vi "Keithley2400_TestReadout&Reset.vi"() -> ()   [LabVIEW 2018]
uses:
  <instrlib>/Keithley 24XX/Public/Data/Read (Single Point).vi
  <instrlib>/Keithley 24XX/Keithley 24XX.lvlib
panel:
  in  "Reset (Note, you  may need to set TRUE to get readout working! \nDon't use TRUE when measuring a device!). This program should loop\nthe voltage from the sourcemeter from 0V to 0.5V then jump to 0V and repeat.":bool
  in  "stop":bool
  out "Interal Measurement Time":u32
  out "Voltage vs N : XYGraph 2":cluster{"Y":dbl[], "Y":dbl[]}[](graph)
  out "Gate\nVoltage":sgl
  out "Status":sgl
  out "Leakage \nCurrent":sgl
  out "I_leak vs N : XYGraph":cluster{"Y":dbl[], "Y":dbl[]}[](graph)
  out "Compliance\n Level (A)":dbl=0.1
  in  "Serial Configuration":T1={"Baud Rate"=9600, "Parity"=0, "Data Bits"=8, "Stop Bits"=10, "Flow Control"=0} {"Flow Control" items=["None", "XON/XOFF", "RTS/CTS", "XON/XOFF & RTS/CTS", "DTR/DSR", "XON/XOFF & DTR/DSR"]; "Stop Bits" items=["1.0"=10, "1.5"=15, "2.0"=20]; "Data Bits" items=["7"=7, "8"=8]; "Parity" items=["None", "Odd", "Even", "Mark", "Space"]; "Baud Rate" items=["300"=300, "600"=600, "1200"=1200, "2400"=2400, "4800"=4800, "9600"=9600, "19200"=19200]}
  in  "Keithley24XX VISA resource name":refnum<visa-resource-name>="GPIB0::21::INSTR" caption="Keithley 24XX VISA resource name"
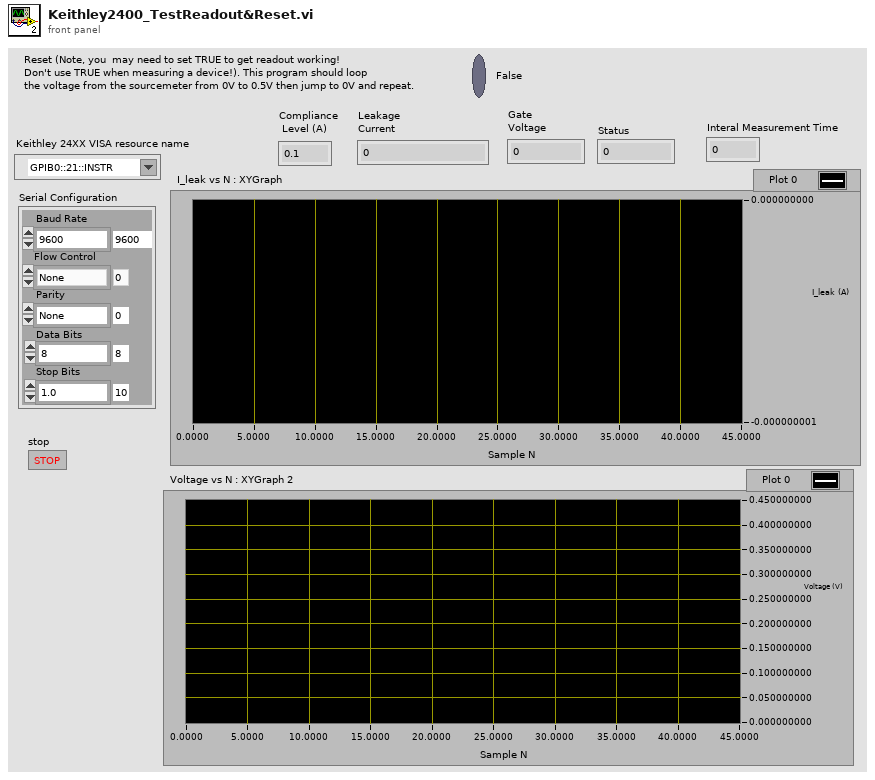
[diagram p1: front panel]
types:
  T1 = cluster{"Baud Rate":u32, "Parity":u16, "Data Bits":u16, "Stop Bits":u16, "Flow Control":u16}
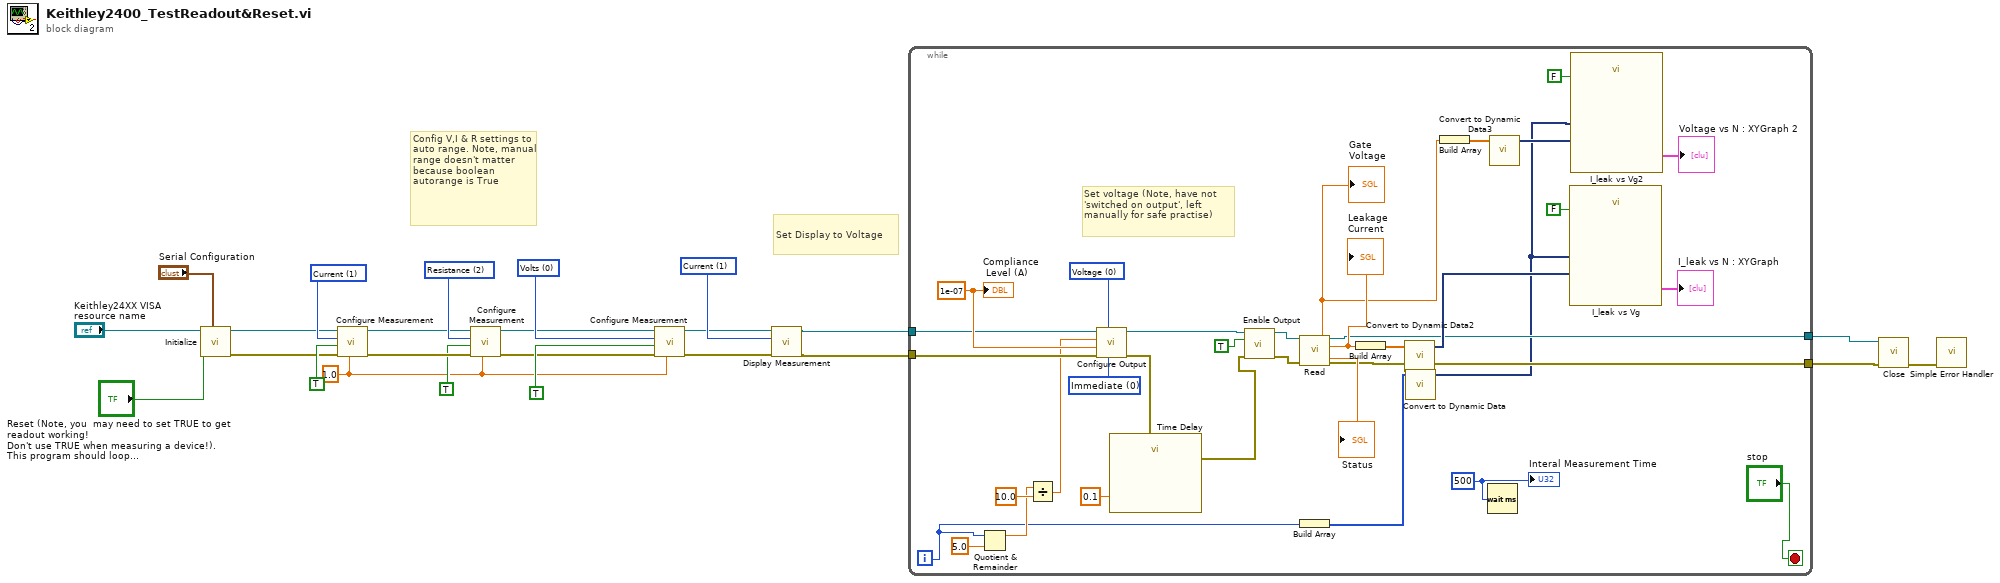
[diagram p0: block diagram]
diagram:
  w7 = 1.0 ("Manual Range (1.0)")
  w11 = u16 1 items=["Voltage", "Current", "Resistance"] ("Displayed Measurement (0: Voltage)")
  w17 = u16 2 items=["Volts", "Current", "Resistance"] ("Function (0: Volts)")
  w21 = u16 1 items=["Volts", "Current", "Resistance"] ("Function (0: Volts)")
  w23 = u16 0 items=["Volts", "Current", "Resistance"] ("Function (0: Volts)")
  # "Set Display to Voltage"
  # "Config V,I & R settings to auto range. Note, manual range doesn't matter because boolean autorange is True"
  n1 = call <instrlib>:"Initialize.vi"("Serial Configuration"="Serial Configuration", "Reset (True)"="Reset (Note, you  may need to set TRUE to get readout working! \nDon't use TRUE when measuring a device!). This program should loop\nthe voltage from the sourcemeter from 0V to 0.5V then jump to 0V and repeat.", "VISA resource name"="Keithley24XX VISA resource name") -> ("error out"=w12:errorcluster, "VISA resource name out"=w13:refnum<visa-resource-name>)  [unwired: 7 in]
  n2 = call <instrlib>:"Configure Measurement.vi"("Manual Range (1.0)"=w7, "error in (no error)"=w12, "Enable Auto Range (T:Enable)"=TRUE, "Function (0: Volts)"=w21, "VISA resource name"=w13) -> ("error out"=w19:errorcluster, "VISA resource name out"=w14:refnum<visa-resource-name>)  [unwired: 5 in]
  n3 = call <instrlib>:"Configure Measurement.vi"("Manual Range (1.0)"=w7, "error in (no error)"=w19, "Enable Auto Range (T:Enable)"=TRUE, "Function (0: Volts)"=w17, "VISA resource name"=w14) -> ("error out"=w16:errorcluster, "VISA resource name out"=w15:refnum<visa-resource-name>)  [unwired: 5 in]
  n4 = call <instrlib>:"Configure Measurement.vi"("Manual Range (1.0)"=w7, "error in (no error)"=w16, "Enable Auto Range (T:Enable)"=TRUE, "Function (0: Volts)"=w23, "VISA resource name"=w15) -> ("error out"=w9:errorcluster, "VISA resource name out"=w10:refnum<visa-resource-name>)  [unwired: 5 in]
  n5 = call <instrlib>:"Display Measurement.vi"("error in (no error)"=w9, "Displayed Measurement (0: Voltage)"=w11, "VISA resource name"=w10) -> ("error out"=w5:errorcluster, "VISA resource name out"=w6:refnum<visa-resource-name>)  [unwired: 7 in]
  n6 = while {
    tunnel: w6 -> [w45]
    tunnel: w5 -> [w44]
    tunnel: [w36] -> w3
    tunnel: [w35] -> w2
    i -> [w37]
    stop <- "stop" stop-if-true
    w31 = u32 500 ("milliseconds to wait")
    w49 = u16 0 items=["Immediate", "Triggered"] ("Output Type  (0: Immediate)")
    w58 = 1e-07 ("Compliance  Level (0.1)")
    w54 = u16 0 items=["Voltage", "Current"] ("Source Mode  (0: Voltage)")
    # "Set voltage (Note, have not 'switched on output', left manually for safe practise)"
    n7 = Quotient & Remainder(x=w37, y=5.0) -> (x-y*floor(x/y)=w40:dbl)  [unwired: 1 out]
    n8 = Divide(x=w40, y=10.0) -> (x/y=w39:dbl)
    n9 = call <instrlib>:"Configure Output.vi"("Output Type  (0: Immediate)"=w49, "Source Mode  (0: Voltage)"=w54, "error in (no error)"=w44, "Compliance  Level (0.1)"=w58, "Output Level (0)"=w39, "VISA resource name"=w45) -> ("error out"=w43:errorcluster, "VISA resource name out"=w57:refnum<visa-resource-name>)  [unwired: 4 in]
    n10 = call "Time Delay"("error in (no error)"=w43, "Delay Time (s)"=0.1) -> ("error out"=w48:errorcluster)  [unwired: 9 in]
    n11 = call <instrlib>:"Enable Output.vi"("error in (no error)"=w48, "Enable Output (T: Enable)"=TRUE, "VISA resource name"=w57) -> ("error out"=w56:errorcluster, "VISA resource name out"=w55:refnum<visa-resource-name>)  [unwired: 7 in]
    n12 = call-poly <instrlib>:"Read.vi"("VISA resource name"=w55, "error in (no error)"=w56) -> ("Voltage"=w32:sgl, "VISA resource name out"=w36:refnum<visa-resource-name>, "Current"=w47:sgl, "Status"=→"Status":sgl, "error out"=w35:errorcluster)  [unwired: 7 in, 2 out]
    "Leakage \nCurrent" <- w47
    "Gate\nVoltage" <- w32
    n13 = Build Array(w37) -> (w38:i32[])
    n14 = Build Array(w47) -> (w51:sgl[])
    n15 = call "Convert to Dynamic Data2"("Array"=w51) -> ("Dynamic Data Type"=w50:dynamicdata)  [unwired: 3 in]
    n16 = call "Convert to Dynamic Data"("Array"=w38) -> ("Dynamic Data Type"=w28:dynamicdata)  [unwired: 3 in]
    n17 = Build Array(w32) -> (w33:sgl[])
    n18 = Wait (ms)(milliseconds to wait=w31) -> ()  [unwired: 1 out]
    n19 = call "Convert to Dynamic Data3"("Array"=w33) -> ("Dynamic Data Type"=w29:dynamicdata)  [unwired: 3 in]
    n20 = call "I_leak vs Vg"("Reset"=FALSE, "Y Input"=w50, "X Input"=w28) -> ("XY Graph"=→"I_leak vs N : XYGraph":cluster{"X":dbl[], "Y":dbl[]}[])  [unwired: 7 in, 1 out]
    n21 = call "I_leak vs Vg2"("Reset"=FALSE, "Y Input"=w29, "X Input"=w28) -> ("XY Graph"=→"Voltage vs N : XYGraph 2":cluster{"X":dbl[], "Y":dbl[]}[])  [unwired: 7 in, 1 out]
    "Compliance\n Level (A)" <- w58
    "Interal Measurement Time" <- w31
  }
  n22 = call <instrlib>:"Close.vi"("error in (no error)"=w2, "VISA resource name"=w3) -> ("error out"=w4:errorcluster)  [unwired: 9 in]
  n23 = call <vilib>:"Simple Error Handler.vi"("error in (no error)"=w4) -> ()  [unwired: 4 in, 5 out]
